vi "SubVIForAsynchronousCall.vi"(8 "error in (no error)":errorcluster) -> (0 "error out":errorcluster)   [LabVIEW 2013]
panel:
  out "Loop":i32
  in  "Exit":bool
  # "§Ú¬O¡@¢á¢ã¢Ð¡@¢ä¢×\nFor Asynchronous Call"
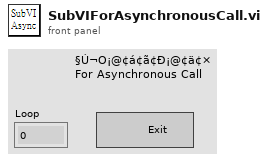
[diagram p1: front panel]
types:
  T1 = enum32{"Invalid", "Standard", "Closed", "Hidden", "Minimized", "Maximized"}
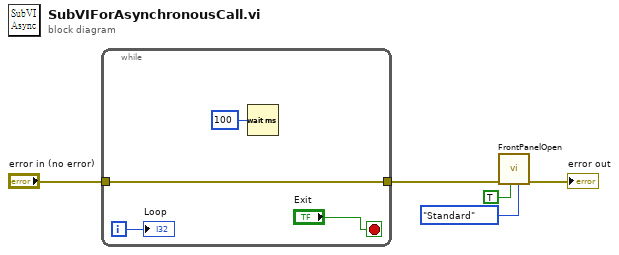
[diagram p0: block diagram]
diagram:
  n1 = while {
    tunnel: [w7] -> w2
    tunnel: "error in (no error)" -> [w7]
    i -> [w6]
    stop <- "Exit" stop-if-true
    n2 = Wait (ms)(milliseconds to wait=u32 100) -> ()  [unwired: 1 out]
    "Loop" <- w6
  }
  n3 = call "FrontPanelOpen.vi"("State"=T1."Standard", "Activate?"=TRUE, "error in (no error)"=w2) -> ("error out"=→"error out":errorcluster)  [unwired: 7 in, 1 out]
